vi "runFirstState.vi"(6 "Fault?":bool, 7 "Ready":bool, 8 "error in (no error)":errorcluster, 9 "Actuators in":T1, 10 "State in":T2, 11 "SystemsCheck in":refnum<class "SystemsCheck.lvclass">) -> (0 "error out":errorcluster, 1 "Actuators out":T1, 2 "State out":T2, 3 "SystemsCheck out":refnum<class "SystemsCheck.lvclass">)   [LabVIEW 2018, in "ControlLibrary.lvlib" / "SystemsCheck.lvclass"]
uses:
  SystemsCheck.lvclass
  TypeDef_ControlState.ctl
  TypeDef_DigitalOuts.ctl
  RunTypeList.ctl
  RunTypeClass/RunType.lvclass
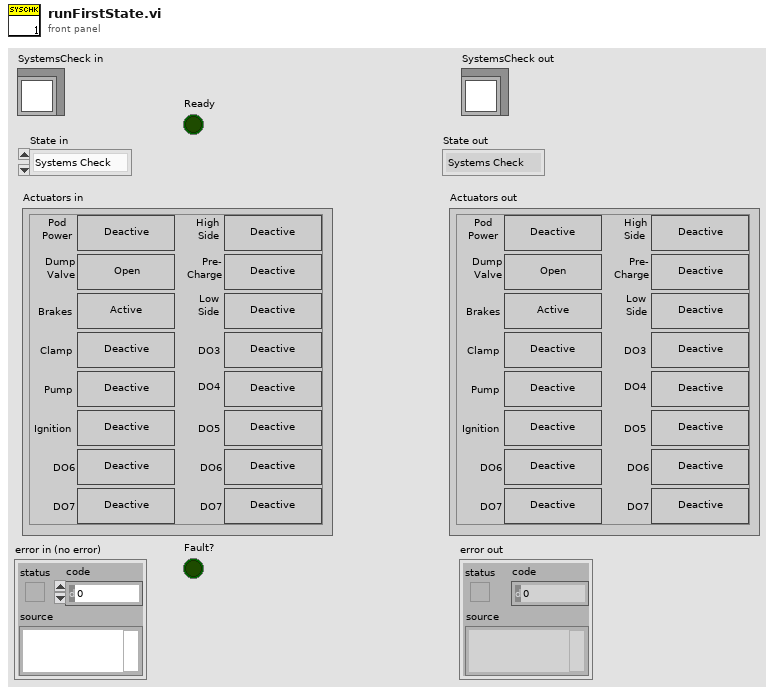
[diagram p1: front panel]
types:
  T1 = typedef "TypeDef_DigitalOuts.ctl" = cluster{"Pod Power":bool, "Dump Valve":bool, "Brakes":bool, "Clamp":bool, "Pump":bool, "Ignition":bool, "DO6":bool, "DO7":bool, "HighSide":bool, "Precharge":bool, "LowSide":bool, "DO3":bool, "DO4":bool, "DO5":bool, "DO62":bool, "DO72":bool}
  T2 = typedef "TypeDef_ControlState.ctl" = enum16{"Systems Check", "Idle", "Ready", "Pushing", "Coast", "Braking", "Fault", "Shutdown", "Service", "Precharge", "Blank"}
  T3 = typedef "RunTypeList.ctl" = enum16{"Full Run", "Systems Check", "Service"}
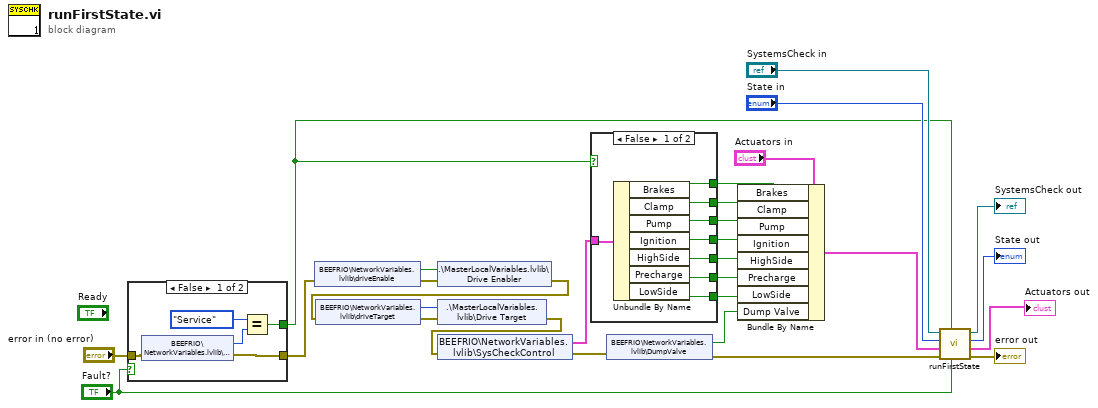
[diagram p0: block diagram]
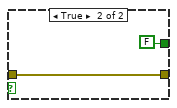
[diagram p2: hidden frame]
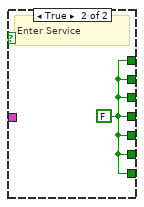
[diagram p3: hidden frame]
diagram:
  n1 = case shown="False" "Fault?" {
    tunnel: "error in (no error)" -> [w32 w35]
    tunnel: [w31 w35] -> w1
    tunnel: [w30 FALSE] -> w20
    frame False {
      n2 = shared-variable "BEEFRIO\\NetworkVariables.lvlib\\RunType"(error in=w32) -> (w34:T3, error out=w31:errorcluster)
      n3 = Equal?(x=RunTypeList."Service", y=w34) -> (x = y?=w30:bool)
    }
    frame True {
    }
  }
  n4 = shared-variable "BEEFRIO\\NetworkVariables.lvlib\\driveEnable"(error in=w1) -> (w5:bool, error out=w4:errorcluster)
  n5 = shared-variable ".\\MasterLocalVariables.lvlib\\Drive Enabler"(w5, error in=w4) -> (error out=w3:errorcluster)
  n6 = shared-variable "BEEFRIO\\NetworkVariables.lvlib\\driveTarget"(error in=w3) -> (w7:i16, error out=w6:errorcluster)
  n7 = shared-variable ".\\MasterLocalVariables.lvlib\\Drive Target"(w7, error in=w6) -> (error out=w2:errorcluster)
  n8 = shared-variable "BEEFRIO\\NetworkVariables.lvlib\\SysCheckControl"(error in=w2) -> (w8:T1, error out=w18:errorcluster)
  n9 = case shown="False" w20 {
    tunnel: [w43 w45] -> w23
    tunnel: [w44 w45] -> w22
    tunnel: [w42 w45] -> w13
    tunnel: [w41 w45] -> w12
    tunnel: [w40 w45] -> w11
    tunnel: [w39 w45] -> w10
    tunnel: [w38 w45] -> w9
    tunnel: w8 -> [w37 _]
    frame False {
      n10 = Unbundle By Name(w37) -> ("Brakes"=w44:bool, "Clamp"=w43:bool, "Pump"=w42:bool, "Ignition"=w41:bool, "HighSide"=w40:bool, "Precharge"=w39:bool, "LowSide"=w38:bool)
    }
    frame True {
      w45 = FALSE
      # "Enter Service"
    }
  }
  n11 = shared-variable "BEEFRIO\\NetworkVariables.lvlib\\DumpValve"(error in=w18) -> (w16:bool, error out=w17:errorcluster)
  n12 = Bundle By Name(cluster="Actuators in", "Brakes"=w22, "Clamp"=w23, "Pump"=w13, "Ignition"=w12, "HighSide"=w11, "Precharge"=w10, "LowSide"=w9, "Dump Valve"=w16) -> (w21:T1)
  n13 = call-parent "runFirstState.vi"("Fault?"="Fault?", "Ready"=w20, "error in (no error)"=w17, "Actuators in"=w21, "State in"="State in", "RunType in"="SystemsCheck in") -> ("error out"=→"error out":errorcluster, "Actuators out"=→"Actuators out":T1, "State out"=→"State out":T2, "RunType out"=→"SystemsCheck out":refnum<class "SystemsCheck.lvclass">)  [unwired: 2 in]
